vi "set_material_on_final_thickness.vi"(8 "error in (no error)":errorcluster, 9 "On final thickness action":T1(ring), 10 "Material number":u8, 11 "VISA resource name":refnum<visa-resource-name>) -> (0 "error out":errorcluster, 3 "VISA resource name out":refnum<visa-resource-name>)   [LabVIEW 2018, in "Inficon IC6.lvlib"]
doc: "Set the state to enter upon reaching the final thickness."
uses:
  <instrlib>/Inficon IC6/Inficon IC6.lvlib
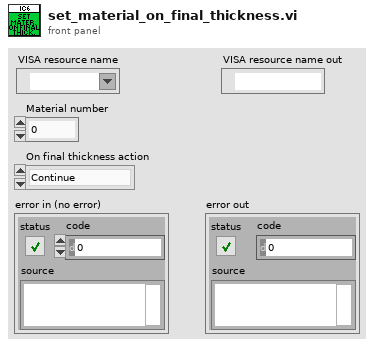
[diagram p1: front panel]
types:
  T1 = enum16{"Continue", "Post-deposit", "Non-deposit control"}
  T2 = enum16{"Source", "General", "Input name", "Process name", "Logic", "Material", "Material name", "Output name", "Process", "Sensor", "Output type", "User message", "Layer", ""}
  T3 = enum16{"Hello", "Query", "Remote action", "Status", "Update"}
  T4 = cluster{"Material number":u8, "On final thickness action":enum16{"Continue", "Post-deposit", "Non-deposit control"}}
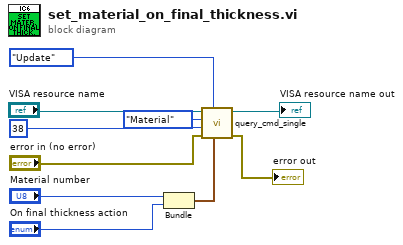
[diagram p0: block diagram]
diagram:
  n1 = Bundle("Material number"="Material number", "On final thickness action"="On final thickness action") -> (w4:T4)  [unwired: 1 in]
  n2 = call <instrlib>:"query_cmd_single.vi"("Parameter"=w4, "Command group"=T3."Update", "error in (no error)"="error in (no error)", "Command ID"=u8 38, "Command subgroup"=T2."Material", "VISA resource name"="VISA resource name") -> ("error out"=→"error out":errorcluster, "VISA resource name out"=→"VISA resource name out":refnum<visa-resource-name>)  [unwired: 1 in, 3 out]
